vi "Enque(AC d).vi"(7 "at front (F)":bool, 8 "error in":errorcluster, 9 "d Cmd Payload":T1, 10 "Message Command":string, 11 "Message que":T4) -> (0 "error out":errorcluster, 3 "Message que out":T4)   [LabVIEW 2019]
doc: "Transmit a message with a waveform array payload.\nFor a regular message, enqueue the message. For a priority message, enqueue it at the front of the queue.\n\nBolder Software LLC"
uses:
  MessageQue/MessageQue.ctl
  MessageQue/MessageCluster.ctl
  Classes/Datalog/DatalogSubvis/SearchableTag.ctl
  Classes/Sequence/SequenceSubvis/RF Direction.ctl
  Classes/Sequence/SequenceSubvis/PolarizationSelect.ctl
  MessageQue/MessageQue.lvlib
  Classes/Datalog/DataLog.lvclass
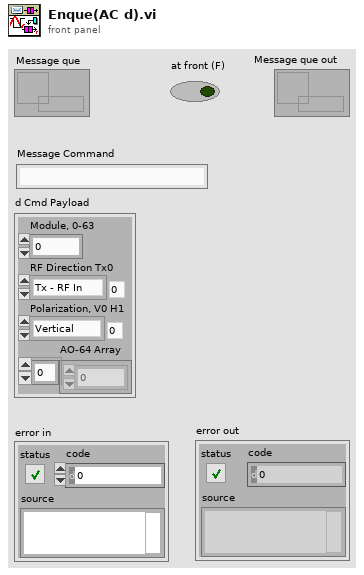
[diagram p1: front panel]
types:
  T1 = typedef "DataLog.lvclass/SearchableTag.ctl" = cluster{"Module, 0-63":i32, "RF Direction Tx0":T2, "Polarization, V0 H1":T3, "AO-64 Array":dbl[]}
  T2 = typedef "RF Direction.ctl" = enum16{"Tx - RF In", "Rx - RF Out"}
  T3 = typedef "PolarizationSelect.ctl" = enum16{"Vertical", "Horizontal"}
  T4 = typedef "MessageQue.lvlib/MessageQue.ctl" = refnum<queue>
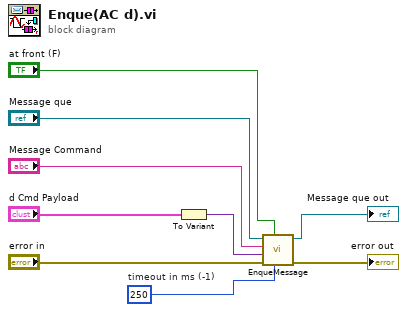
[diagram p0: block diagram]
diagram:
  w9 = 250  # timeout in ms (-1)
  n1 = To Variant(anything="d Cmd Payload") -> (Variant=w3:variant)
  n2 = call "EnqueMessage.vi"("timeout in ms (-1)"=w9, "Priority Message? (F)"="at front (F)", "error in"="error in", "Message Payload"=w3, "Message Command"="Message Command", "Message que"="Message que") -> ("error out"=→"error out":errorcluster, "Message que out"=→"Message que out":T4)  [unwired: 4 in]
